vi "KTable Write Test.vi"() -> ()   [LabVIEW 2015, in "KTable.xctl"]
uses:
  KTable.xctl
  ColumnType.ctl
  ColumnSpec.ctl
panel:
  in  "ColType":T1
  out "Table Items":string[][](array[string])
  in  "Array":cluster{"Val1":string, "Val2":i32, "Val3":T1}[](array[cluster])
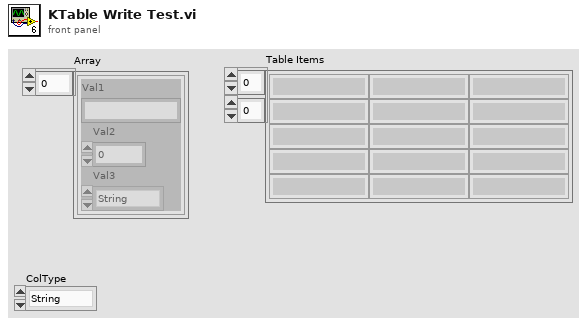
[diagram p1: front panel]
types:
  T1 = typedef "KTable.xctl/ColumnType.ctl" = enum16{"String", "Enum", "Int", "Double", "Boolean", "Ring", "Formula", "Color"}
  T2 = typedef "KTable.xctl/ColumnSpec.ctl" = cluster{"Name":string, "Type":T1, "Width":i32, "Strings":string[], "Position":enum16{"Left", "Center", "Right"}, "locked":bool, "cds":cluster{"Strings":string[]}[][], "Hide NaN":bool}
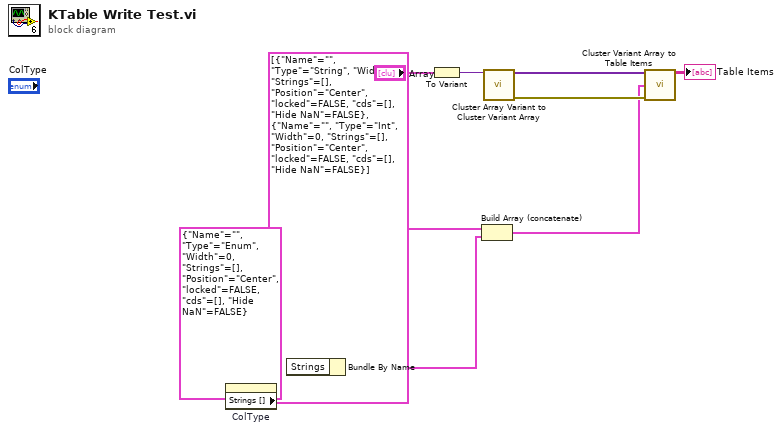
[diagram p0: block diagram]
diagram:
  n1 = property on="ColType" class="Enum (strict)"() -> ("Strings []"=w5:string[])  [unwired: 2 in, 2 out]
  n2 = Bundle By Name(cluster=T2 {"Name"="", "Type"=enum."Enum", "Width"=0, "Strings"=[], "Position"=enum."Center", "locked"=FALSE, "cds"=[], "Hide NaN"=FALSE} ("ColSpec"), "Strings"=w5) -> (w4:T2)
  n3 = To Variant(anything="Array") -> (Variant=w1:variant)
  n4 = Build Array (concatenate)(T2[] [{"Name"="", "Type"=enum."String", "Width"=0, "Strings"=[], "Position"=enum."Center", "locked"=FALSE, "cds"=[], "Hide NaN"=FALSE}, {"Name"="", "Type"=enum."Int", "Width"=0, "Strings"=[], "Position"=enum."Center", "locked"=FALSE, "cds"=[], "Hide NaN"=FALSE}] ("Array"), w4) -> (w2:T2[])
  n5 = call "Cluster Array Variant to Cluster Variant Array.vi"("Variant"=w1) -> ("Array"=w9:variant[], "error out"=w7:errorcluster)  [unwired: 13 in]
  n6 = call "Cluster Variant Array to Table Items.vi"("Cluster Variant Array"=w9, "Columns"=w2, "error in (no error)"=w7) -> ("Table Items"=→"Table Items":string[][])  [unwired: 10 in, 2 out]
